vi "ProdaNG.Convert.I32-U8[].vi"(11 "32bit integer":i32) -> (3 "unsigned byte array":u8[](array[numeric]))   [LabVIEW 2016]
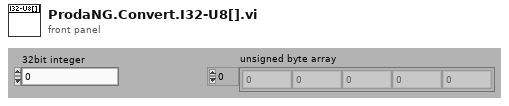
[diagram p1: front panel]
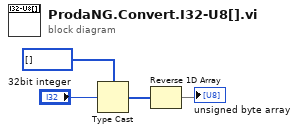
[diagram p0: block diagram]
diagram:
  n1 = Type Cast(type=u8[] [] ("unsigned byte array"), x="32bit integer") -> (*(type *) &x=w2:u8[])
  n2 = Reverse 1D Array(array=w2) -> (reversed array=→"unsigned byte array":u8[])
